vi "CRYDelete All Complete.vi"(11 "sAction":string="XY") -> (1 "Delete?":bool=TRUE, 2 "Deleted Rows":i32[](array[numeric]))   [LabVIEW 2013]
uses:
  CRYSystem/Typedef Control/CRYData Cluster.ctl
  CRYSystem/Typedef Control/CRYResult Cluster.ctl
  CRYSystem/Typedef Control/CRYWaveform Cluster.ctl
panel:
  # "Delete  Data"
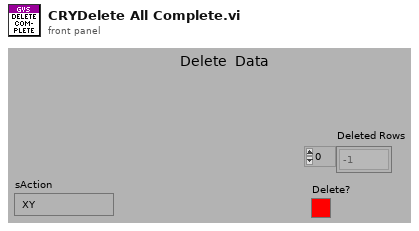
[diagram p1: front panel]
types:
  T1 = typedef "CRYWaveform Cluster.ctl" = cluster{"Waveform":cluster{"X0":dbl, "dX":dbl, "Y":sgl[]}, "X data":u16, "Y data":u16, "Y axis":u16, "X unit":string, "Y unit":string, "Y dB ref":dbl, "display Y":bool, "display X":bool, "Overload?":bool, "Test Info":string, "Step No.":i32, "Name":string, "protected":bool, "Sqc history":string[], "Signal Channel ID":i32, "Plot Settings":cluster{"Color":u32, "Interpolation":u8, "Point Style":u8, "Line Style":u8, "Point Color":u32, "Line Width":u8, "Bar Plot Style":u8, "Fill To":i16}, "AutoProtect":bool}
  T2 = typedef "CRYResult Cluster.ctl" = cluster{"Name":string, "Margin":dbl, "unit":string, "Verdict":bool, "Limit":string, "Max/Min":string, "protected":bool, "Step No.":i32, "Test Info":string, "AutoProtect":bool}
  T3 = typedef "CRYData Cluster.ctl" = cluster{"Name":string, "Curve":cluster{"x":dbl, "y":dbl, "z":dbl}[], "X data":u16, "Y data":u16, "Z data":u16, "X axis":u16, "Y axis":u16, "Z axis":u16, "X unit":string, "Y unit":string, "Z unit":string, "X dB ref":dbl, "Y dB ref":dbl, "Z dB ref":dbl, "single val":bool, "protected":bool, "display X":bool, "display Y":bool, "display Z":bool, "Test Info":string, "Step No.":i32, "Plot Settings":cluster{"Color":u32, "Interpolation":u8, "Point Style":u8, "Line Style":u8, "Point Color":u32, "Line Width":u8, "Bar Plot Style":u8, "Fill To":i16}, "AutoProtect":bool}
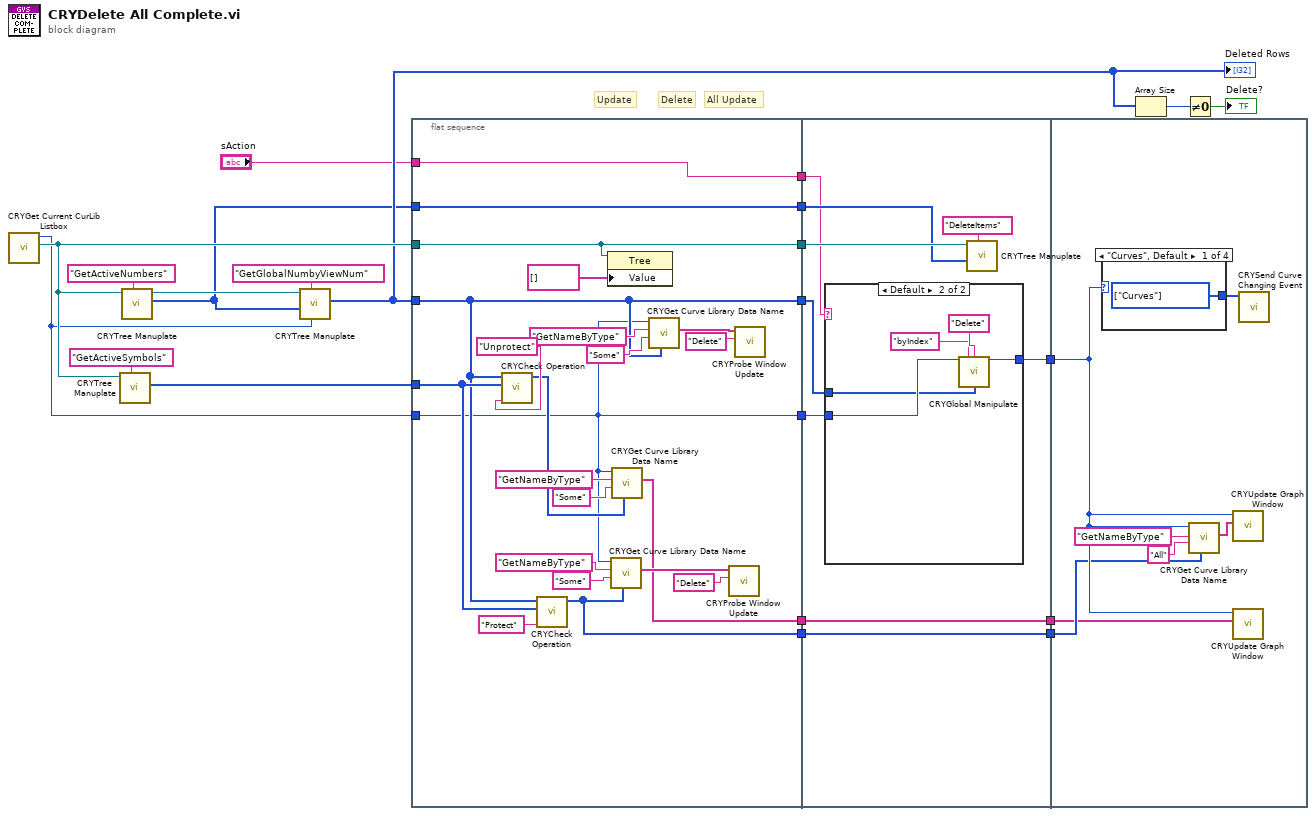
[diagram p0: block diagram]
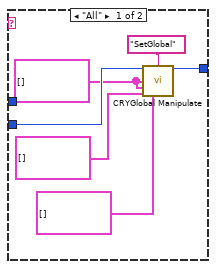
[diagram p2: hidden frame]
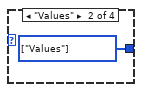
[diagram p3: hidden frame]
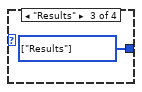
[diagram p4: hidden frame]
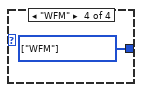
[diagram p5: hidden frame]
diagram:
  # "All Update"
  # "Delete"
  # "Update"
  n1 = call "CRYGet Current CurLib Listbox.vi"() -> ("CurLib Tree"=w15:refnum<vi>, "Type"=w3:enum16{"Curves", "Values", "Results", "WFM"})  [unwired: 9 in, 1 out]
  n2 = call "CRYTree Manuplate.vi"("sAction"="GetActiveSymbols", "Tree in"=w15) -> ("nData Out"=w14:i32[])  [unwired: 6 in, 3 out]
  n3 = call "CRYTree Manuplate.vi"("sAction"="GetActiveNumbers", "Tree in"=w15) -> ("nData Out"=w4:i32[], "Tree Out"=w7:refnum<vi>)  [unwired: 6 in, 2 out]
  n4 = call "CRYTree Manuplate.vi"("Type"=w3, "sAction"="GetGlobalNumbyViewNum", "nData"=w4, "Tree in"=w7) -> ("nData Out"=w6:i32[])  [unwired: 4 in, 3 out]
  "Deleted Rows" <- w6
  n5 = flat-sequence {
    tunnel: w3 -> [w26]
    tunnel: w6 -> [w28]
    tunnel: w15 -> [w25]
    tunnel: [w25] -> w20
    tunnel: [w28] -> w19
    tunnel: [w26] -> w18
    tunnel: w14 -> [w38]
    tunnel: [w30] -> w11
    tunnel: [w29] -> w9
    tunnel: [w27] -> w5
    tunnel: w4 -> [w27]
    tunnel: [w23] -> w2
    tunnel: "sAction" -> [w23]
    tunnel: w20 -> [w48]
    tunnel: w19 -> [w45]
    tunnel: w18 -> [w49]
    tunnel: [w52] -> w13
    tunnel: [w51] -> w12
    tunnel: w11 -> [w51]
    tunnel: [w50] -> w10
    tunnel: w9 -> [w50]
    tunnel: w5 -> [w47]
    tunnel: w2 -> [w46]
    tunnel: w13 -> [w67]
    tunnel: w12 -> [w66]
    tunnel: w10 -> [w65]
    frame #0 {
      n6 = call "CRYCheck Operation.vi"("Operation"="Unprotect", "Item Symbols In"=w38, "Index Array In"=w28) -> ("Array Out"=w37:i32[])  [unwired: 6 in, 2 out]
      n7 = call "CRYCheck Operation.vi"("Operation"="Protect", "Item Symbols In"=w38, "Index Array In"=w28) -> ("Array Out"=w30:i32[])  [unwired: 6 in, 2 out]
      n8 = property class="Tree"(reference=w25, "Value"=string[] [] ("sNames")) -> ()  [unwired: 1 in, 2 out]
      n9 = call "CRYGet Curve Library Data Name.vi"("nData"=w30, "sOption"="Some", "sAction"="GetNameByType", "Type"=w26) -> ("sNames"=w43:string[])  [unwired: 2 in, 5 out]
      n10 = call "CRYGet Curve Library Data Name.vi"("nData"=w37, "sOption"="Some", "sAction"="GetNameByType", "Type"=w26) -> ("sNames"=w29:string[])  [unwired: 2 in, 5 out]
      n11 = call "CRYGet Curve Library Data Name.vi"("nData"=w28, "sOption"="Some", "sAction"="GetNameByType", "Type"=w26) -> ("sNames"=w44:string[])  [unwired: 2 in, 5 out]
      n12 = call "CRYProbe Window Update.vi"("sAction"="Delete", "Names"=w43) -> ()  [unwired: 2 in, 8 out]
      n13 = call "CRYProbe Window Update.vi"("sAction"="Delete", "Names"=w44) -> ()  [unwired: 2 in, 8 out]
    }
    frame #1 {
      n14 = case shown="Default" w46 {
        tunnel: [w58 w63] -> w52
        tunnel: w49 -> [w57 w62]
        tunnel: w45 -> [_ w61]
        frame "All" {
          w56 = T3[] [] ("Curves")
          n15 = call "CRYGlobal Manipulate.vi"("Type"=w57, "sAction"="SetGlobal", "Curves"=w56, "Values"=w56, "Results"=T2[] [], "WFM"=T1[] []) -> ("Type out"=w58:enum16{"Curves", "Values", "Results", "WFM"})  [unwired: 3 in, 6 out]
        }
        frame Default {
          n16 = call "CRYGlobal Manipulate.vi"("Type"=w62, "sOption"="byIndex", "sAction"="Delete", "nData"=w61) -> ("Type out"=w63:enum16{"Curves", "Values", "Results", "WFM"})  [unwired: 5 in, 6 out]
        }
      }
      n17 = call "CRYTree Manuplate.vi"("sAction"="DeleteItems", "nData"=w47, "Tree in"=w48) -> ()  [unwired: 5 in, 4 out]
    }
    frame #2 {
      n18 = case shown="\"Curves\", Default" w67 {
        tunnel: [w72 w73 w74 w75] -> w71
        frame "Curves", Default {
          w72 = enum16{"Curves", "Values", "Results", "WFM"}[] [enum."Curves"] items=["Curves", "Values", "Results", "WFM"] ("Type")
        }
        frame "Values" {
          w73 = enum16{"Curves", "Values", "Results", "WFM"}[] [enum."Values"] items=["Curves", "Values", "Results", "WFM"] ("Type")
        }
        frame "Results" {
          w74 = enum16{"Curves", "Values", "Results", "WFM"}[] [enum."Results"] items=["Curves", "Values", "Results", "WFM"] ("Type")
        }
        frame "WFM" {
          w75 = enum16{"Curves", "Values", "Results", "WFM"}[] [enum."WFM"] items=["Curves", "Values", "Results", "WFM"] ("Type")
        }
      }
      n19 = call "CRYGet Curve Library Data Name.vi"("nData"=w66, "sOption"="All", "sAction"="GetNameByType", "Type"=w67) -> ("sNames"=w70:string[])  [unwired: 2 in, 5 out]
      n20 = call "CRYUpdate Graph Window.vi"("Del/Update Names"=w70, "Type"=w67) -> ()  [unwired: 2 in, 8 out]
      n21 = call "CRYUpdate Graph Window.vi"("Del/Update Names"=w65, "Type"=w67) -> ()  [unwired: 2 in, 8 out]
      n22 = call "CRYSend Curve Changing Event.vi"("Type"=w71) -> ()  [unwired: 11 out]
    }
  }
  n23 = Array Size(array=w6) -> (size(s)=w21:i32)
  n24 = Not Equal To 0?(x=w21) -> (x != 0?=→"Delete?":bool)
